vi "Main.vi"(11 "Module Admin":refnum<class "Delacor_lib_QMH_Module Admin.lvclass">) -> ()   [LabVIEW 2020, in "Config.lvlib"]
doc: "This template is based off of the Queued Message Handler design pattern and the Queued Message Handler project template that ships with LabVIEW.\n\nThe main difference is that the queue is private to this module and communication between modules is performed via Broadcast and Request events.\n\nRequest events are wrapped in public API methods and are handled in the Event Handling Loop (EHL) of this VI. Any module can register for Broadcast events sent by this module. The EHL generates messages based on user interface actions.\n\nThe Message Handling Loop (MHL) processes messages generated by the EHL, or by other messages. The messages are string values, so new messages can be added easily to the Message Cases case structure in the MHL. Each message cluster can also provide an optional value for Message Data, which is a variant that can be converted to whatever message-specific data is required.\n_____\nBased on Delacor QMH Project Template 5.0.0.82."
uses:
  Config.lvlib
  <vilib>/Delacor/Delacor QMH/Libraries/Module Admin_class/Delacor_lib_QMH_Module Admin.lvclass
  Module Data--cluster.ctl
  Stop Argument--cluster.ctl
  <vilib>/Delacor/Delacor QMH/Libraries/Message Queue_class/Delacor_lib_QMH_Message Queue.lvclass/Delacor_lib_QMH_Message Queue.ctl
  <vilib>/Delacor/Delacor QMH/Libraries/Module Admin_class/Delacor_lib_QMH_Module Admin.lvclass/Delacor_lib_QMH_Module Admin.ctl
  <vilib>/Utility/sysdir.llb/System Directory Type.ctl
  <vilib>/Delacor/Delacor QMH/Libraries/Message Queue_class/Delacor_lib_QMH_Enqueue Message (Single).vi
  <vilib>/Delacor/Delacor QMH/Libraries/Module Admin_class/Delacor_lib_QMH_Get External Launch.vi
  <vilib>/Utility/error.llb/Error Cluster From Error Code.vi
  <vilib>/ErrorRing/Error Ring.xnode
  <vilib>/Delacor/Delacor QMH/Libraries/Message Queue_class/Delacor_lib_QMH_Message Queue.lvclass
  Monedas/Monedas.lvlib
  Productos/Productos.lvlib
panel:
  in  "Productos":T1(array[cluster])
  in  "Monedas":cluster{"Valor":dbl, "Visible":bool}[](array[cluster])
  out "error out":errorcluster
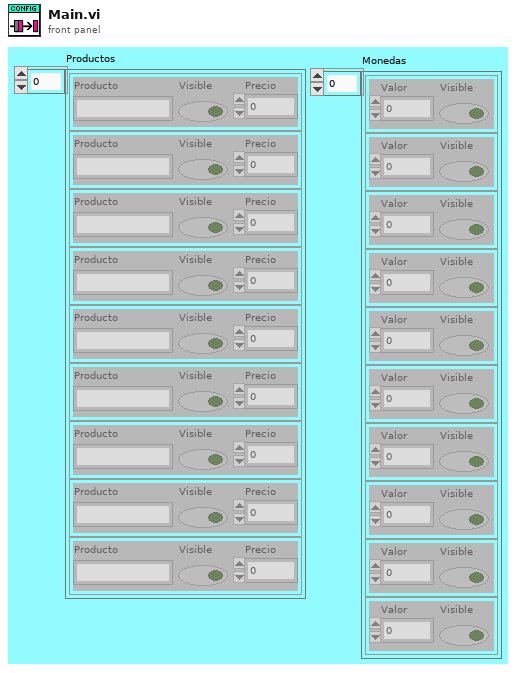
[diagram p1: front panel]
types:
  T1 = cluster{"Producto":string, "Visible":bool, "Precio":dbl}[]
  T2 = typedef "Config.lvlib/Request Events--cluster.ctl" = cluster{"Stop Module":refnum<user-event>, "Show Panel":refnum<user-event>, "Hide Panel":refnum<user-event>, "Get Module Execution Status":refnum<user-event>, "Show Diagram":refnum<user-event>}
  T3 = typedef "Config.lvlib/Module Data--cluster.ctl" = cluster{"Status":string}
  T4 = enum32{"invalid lock state", "Not Locked", "Locked (No Password)", "Password-protected"}
  T5 = typedef "Config.lvlib/Stop Argument--cluster.ctl" = cluster{"Origin":string, "Exit via Stop Module Req?":bool, "Wait for Module to stop?":bool}
  T6 = enum32{"Invalid", "Standard", "Closed", "Hidden", "Minimized", "Maximized"}
  T7 = enum16{"open", "replace", "create", "open or create", "replace or create", "replace or create with confirmation"}
  T8 = cluster{"Producto":string, "Boolean":bool, "Precio":dbl}[]
  T9 = typedef "System Directory Type.ctl" = i32
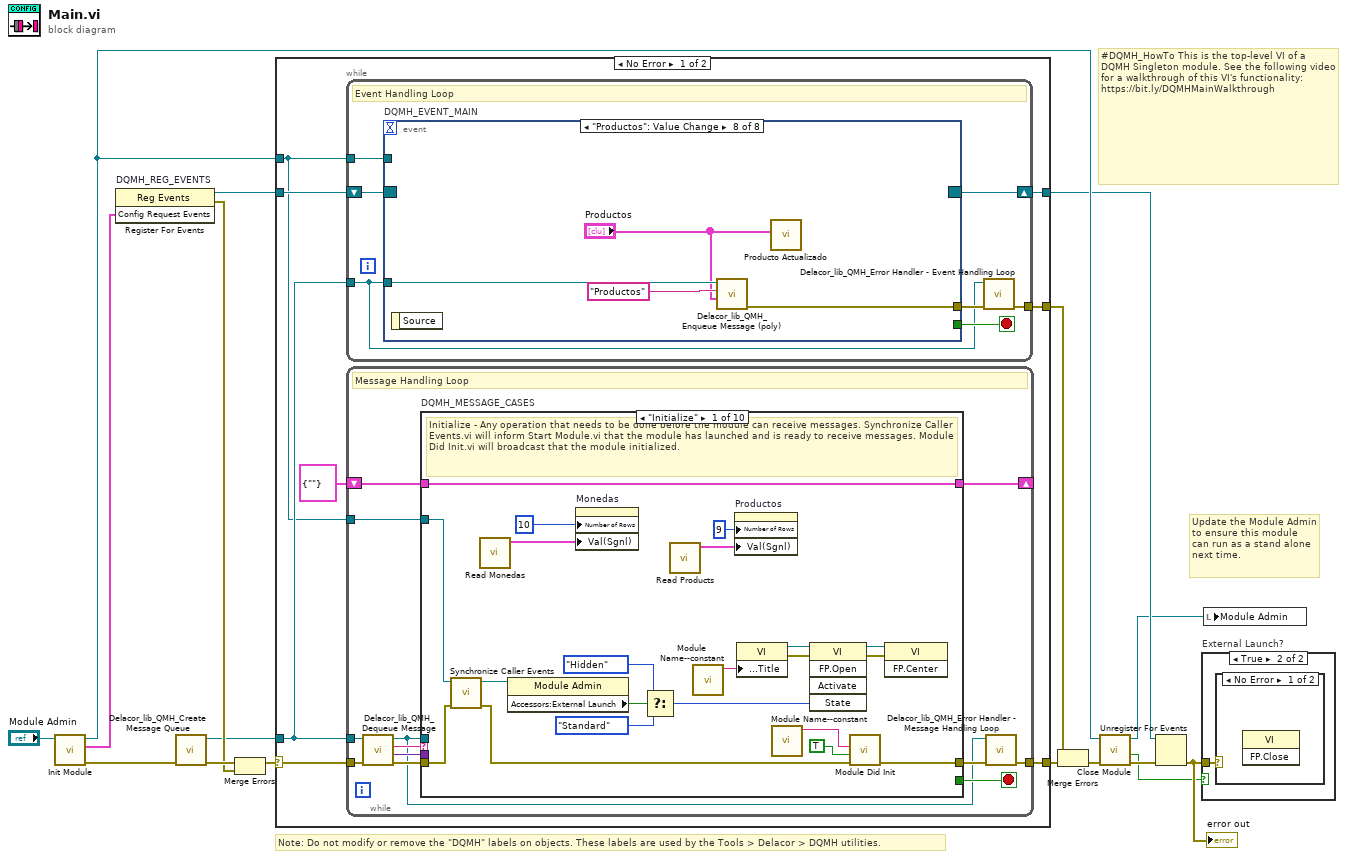
[diagram p0: block diagram]
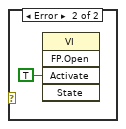
[diagram p3: hidden frame]
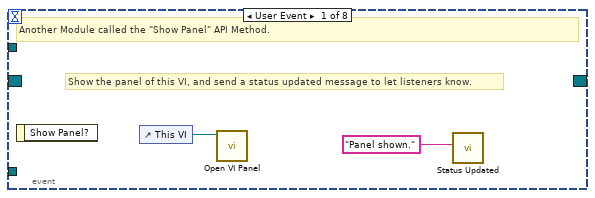
[diagram p4: hidden frame]
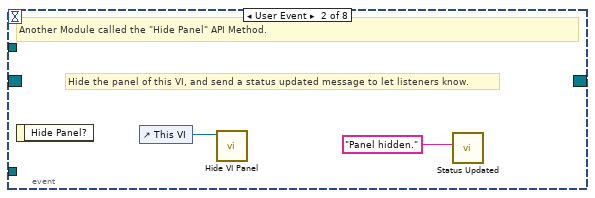
[diagram p5: hidden frame]
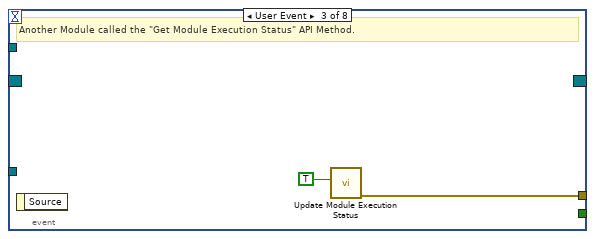
[diagram p6: hidden frame]
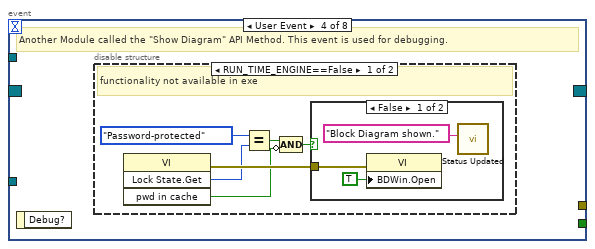
[diagram p7: hidden frame]
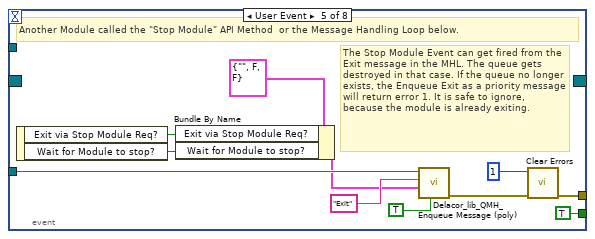
[diagram p10: hidden frame]
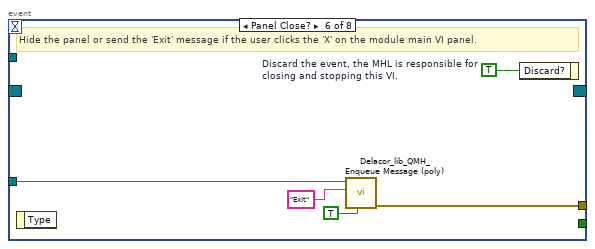
[diagram p11: hidden frame]
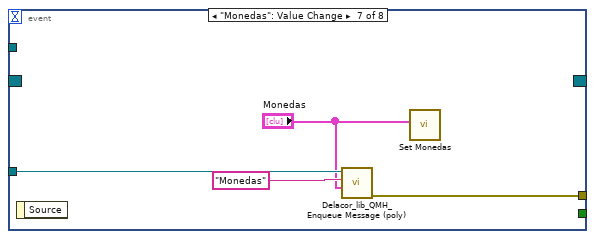
[diagram p12: hidden frame]
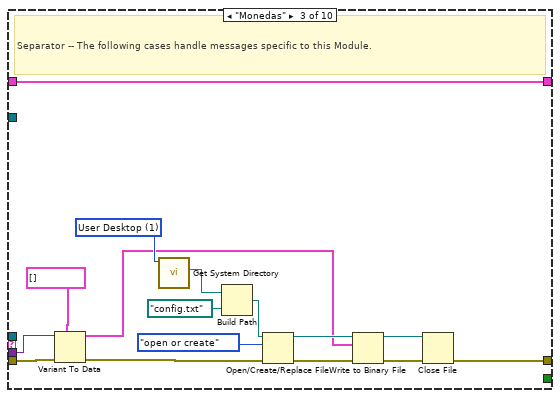
[diagram p14: hidden frame]
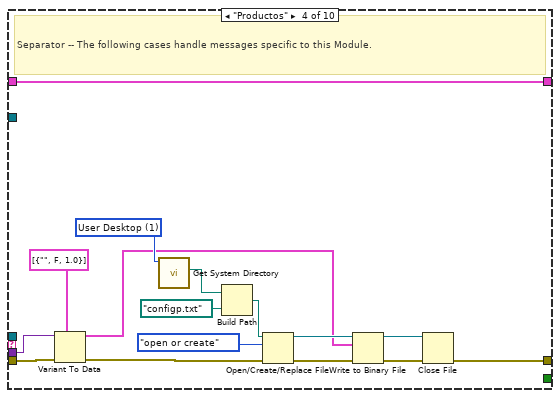
[diagram p15: hidden frame]
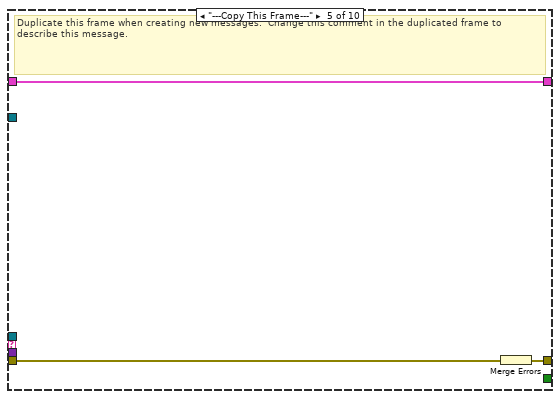
[diagram p16: hidden frame]
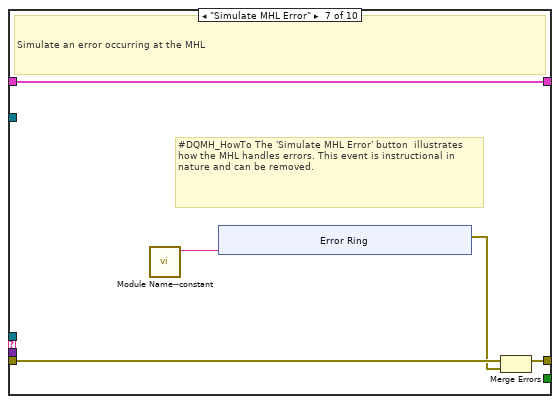
[diagram p18: hidden frame]
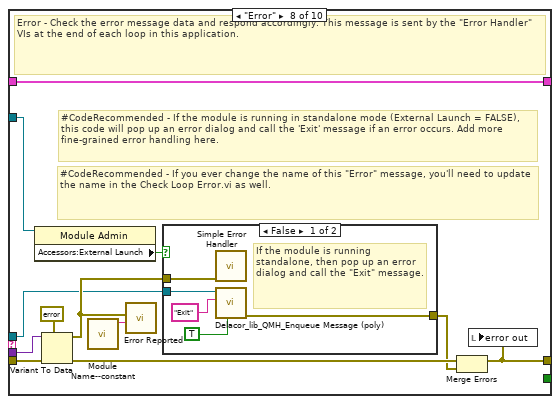
[diagram p19: hidden frame]
diagram:
  # "#DQMH_HowTo This is the top-level VI of a DQMH Singleton module. See the following video for a walkthrough of this VI's functionality: https://bit.ly/DQMHMainWalkthrough"
  # "Note: Do not modify or remove the \"DQMH\" labels on objects. These labels are used by the Tools > Delacor > DQMH utilities."
  # "Update the Module Admin to ensure this module can run as a stand alone next time."
  n1 = call "Init Module.vi"("Singleton Module Admin in"="Module Admin") -> ("error out"=w16:errorcluster, "Config Request Events"=w5:T2, "Singleton Module Admin out"=w8:refnum<class "Delacor_lib_QMH_Module Admin.lvclass">)  [unwired: 8 in]
  n2 = register-events "DQMH_REG_EVENTS"(w5) -> (reference out=w6:refnum<event-registration>, error out=w9:errorcluster)  [unwired: 2 in]
  n3 = call <vilib>:"Delacor_lib_QMH_Create Message Queue.vi"("error in (no error)"=w16) -> ("error out"=w11:errorcluster, "Message Queue"=w4:refnum<class "Delacor_lib_QMH_Message Queue.lvclass">)  [unwired: 9 in]
  n4 = Merge Errors(w11, w9) -> (w10:errorcluster)
  n5 = case shown="No Error" w10 {
    selector: w10 -> [w23 w204]
    tunnel: [w25 w203] -> w17
    tunnel: [w22 w209] -> w7
    tunnel: w6 -> [w20 w209]
    tunnel: w4 -> [w19 w202]
    tunnel: [w24 _] -> w14
    tunnel: w8 -> [w18 w205]
    frame No Error {
      n6 = while {
        tunnel: w19 -> [w26]
        shift-right: [w29] -> w22
        shift-left: w20 -> [w30]
        tunnel: [w31] -> w24
        tunnel: w18 -> [w27]
        stop <- w28 stop-if-true
        # "Event Handling Loop"
        n7 = event "DQMH_EVENT_MAIN" shown="[7] \"Productos\": Value Change" {
          selector: w30 -> [_ _ _ _ _ _ _ _]
          dyn-events: [_ _ _ _ _ _ _ _] -> w29
          timeout: _ -> [_ _ _ _ _ _ _ _]
          tunnel: [_ _ _ _ TRUE ("Discard?") _ _ _] -> w28
          tunnel: w26 -> [_ _ _ _ w54 w61 w66 w70]
          tunnel: [_ _ w38 _ w57 w63 w65 w69] -> w32
          tunnel: w27 -> [_ _ _ _ _ _ _ _]
          event User Event {
            # "Show the panel of this VI, and send a status updated message to let listeners know."
            # "Another Module called the \"Show Panel\" API Method."
            n8 = event-data() -> ()  [unwired: 1 in, 1 out]
            n9 = control-ref of="This VI"() -> (w34:refnum<vi>)
            n10 = call "Open VI Panel.vi"("VI"=w34) -> ()  [unwired: 10 in, 1 out]
            n11 = call "Status Updated.vi"("Status"="Panel shown." ("format string")) -> ()  [unwired: 10 in, 1 out]
          }
          event User Event {
            # "Hide the panel of this VI, and send a status updated message to let listeners know."
            # "Another Module called the \"Hide Panel\" API Method."
            n12 = event-data() -> ()  [unwired: 1 in, 1 out]
            n13 = control-ref of="This VI"() -> (w36:refnum<vi>)
            n14 = call "Hide VI Panel.vi"("VI"=w36) -> ()  [unwired: 10 in, 1 out]
            n15 = call "Status Updated.vi"("Status"="Panel hidden." ("format string")) -> ()  [unwired: 10 in, 1 out]
          }
          event User Event {
            # "Another Module called the \"Get Module Execution Status\" API Method."
            n16 = event-data() -> ()  [unwired: 1 in, 1 out]
            n17 = call "Update Module Execution Status.vi"("Running?"=TRUE) -> ("error out"=w38:errorcluster)  [unwired: 10 in]
          }
          event User Event {
            # "Another Module called the \"Show Diagram\" API Method. This event is used for debugging."
            n18 = event-data() -> ()  [unwired: 1 in, 1 out]
            n19 = disable-structure shown="RUN_TIME_ENGINE==False" {
              frame condition #0 (active) {
                # "functionality not available in exe"
                n20 = invoke class="VI" method="Lock State.Get"() -> (error out=w44:errorcluster, "Get Lock State"=w43:T4, "pwd in cache"=w40:bool)  [unwired: 4 in, 1 out]
                n21 = Equal?(x=T4."Password-protected", y=w43) -> (x = y?=w41:bool)
                n22 = Compound Arithmetic op=AND(w41, invert w40) -> (w39:bool)
                n23 = case shown="False" w39 {
                  tunnel: w44 -> [w47 _]
                  frame False {
                    n24 = property class="VI"(error in=w47, "BDWin.Open"=TRUE ("Block Diagram Window:Open")) -> ()  [unwired: 1 in, 2 out]
                    n25 = call "Status Updated.vi"("Status"="Block Diagram shown." ("format string")) -> ()  [unwired: 10 in, 1 out]
                  }
                  frame True {
                    # "Password-protected VI, and the password is not in the cache. Do not show the diagram."
                  }
                }
              }
              frame condition #1 {
              }
            }
          }
          event User Event {
            # "The Stop Module Event can get fired from the Exit message in the MHL. The queue gets destroyed in that case. If the queue no longer exists, the Enqueue Exit as a priority message will return error 1. It is safe to ignore, because the module is already exiting."
            # "Another Module called the \"Stop Module\" API Method  or the Message Handling Loop below."
            n26 = event-data() -> ("Exit via Stop Module Req?"=w50:bool, "Wait for Module to stop?"=w49:bool)  [unwired: 1 in]
            n27 = Bundle By Name(cluster=T5 {"Origin"="", "Exit via Stop Module Req?"=FALSE, "Wait for Module to stop?"=FALSE} ("Stop Argument"), "Exit via Stop Module Req?"=w50, "Wait for Module to stop?"=w49) -> (w48:T5)
            n28 = call-poly <vilib>:"Delacor_lib_QMH_Enqueue Message (poly).vi"("Priority Message? (F)"=TRUE, "Message Data"=w48, "Message"="Exit", "Message Queue in"=w54) -> ("error out"=w58:errorcluster)  [unwired: 6 in, 1 out]
            n29 = call <vilib>:"Clear Errors.vi"("error in (no error)"=w58, "specific error code to clear (0: all)"=1) -> ("error out"=w57:errorcluster)  [unwired: 4 in, 1 out]
          }
          event Panel Close? {
            w62 = TRUE  # Discard the event, the MHL is responsible for closing and stopping this VI.
            # "Hide the panel or send the 'Exit' message if the user clicks the 'X' on the module main VI panel."
            n30 = event-data() -> ()  [unwired: 1 in, 1 out]
            n31 = call-poly <vilib>:"Delacor_lib_QMH_Enqueue Message (poly).vi"("Priority Message? (F)"=TRUE, "Message"="Exit", "Message Queue in"=w61) -> ("error out"=w63:errorcluster)  [unwired: 7 in, 1 out]
            n32 = event-data("Discard?"=w62) -> ()  [unwired: 1 in, 1 out]
          }
          event "Monedas": Value Change {
            n33 = event-data() -> ()  [unwired: 1 in, 1 out]
            n34 = call-poly <vilib>:"Delacor_lib_QMH_Enqueue Message (poly).vi"("Message Data"="Monedas", "Message"="Monedas", "Message Queue in"=w66) -> ("error out"=w65:errorcluster)  [unwired: 7 in, 1 out]
            n35 = call "Set Monedas.vi"("Monedas"="Monedas") -> ()  [unwired: 10 in, 1 out]
          }
          event "Productos": Value Change {
            n36 = event-data() -> ()  [unwired: 1 in, 1 out]
            n37 = call-poly <vilib>:"Delacor_lib_QMH_Enqueue Message (poly).vi"("Message Data"="Productos", "Message"="Productos", "Message Queue in"=w70) -> ("error out"=w69:errorcluster)  [unwired: 7 in, 1 out]
            n38 = call "Producto Actualizado.vi"("Array"="Productos") -> ()  [unwired: 10 in, 1 out]
          }
        }
        n39 = call-dynamic "Delacor_lib_QMH_Error Handler - Event Handling Loop.vi"("error in (no error)"=w32, "Message Queue in"=w26) -> ("dup error in"=w31:errorcluster)  [unwired: 8 in, 1 out]
      }
      n40 = while {
        tunnel: w19 -> [w74]
        shift-right: [w78] -> _
        shift-left: T3 {"Status"=""} ("Data Cluster") -> [w79]
        tunnel: w23 -> [w82]
        tunnel: [w80] -> w25
        tunnel: w18 -> [w72]
        stop <- w77 stop-if-true
        # "Message Handling Loop"
        n41 = call-dynamic "Delacor_lib_QMH_Dequeue Message.vi"("error in (no error)"=w82, "Message Queue in"=w74) -> ("error out"=w81:errorcluster, "Message Data"=w75:variant, "Message"=w76:string, "Message Queue out"=w73:refnum<class "Delacor_lib_QMH_Message Queue.lvclass">)  [unwired: 6 in]
        n42 = case "DQMH_MESSAGE_CASES" shown="\"Initialize\"" w76 {
          selector: w76 -> [_ _ _ _ _ _ _ _ _ w189]
          tunnel: w73 -> [_ _ _ _ _ _ _ w159 w181 _]
          tunnel: w81 -> [w102 w106 w113 w129 w141 w143 w148 w166 w187 w191]
          tunnel: [w100 w106 w112 w128 w140 w143 w147 w162 w184 w192] -> w83
          tunnel: w79 -> [w91 w105 w122 w138 w139 w142 w145 w161 w180 w190]
          tunnel: [w91 w105 w122 w138 w139 w142 w145 w161 w180 w190] -> w78
          tunnel: [_ _ _ _ _ _ _ _ w179 _] -> w77
          tunnel: w75 -> [_ _ w109 w125 _ _ _ w160 w178 _]
          tunnel: w72 -> [w92 _ _ _ _ _ _ w158 w173 _]
          frame "Initialize" {
            # "Initialize - Any operation that needs to be done before the module can receive messages. Synchronize Caller Events.vi will inform Start Module.vi that the module has launched and is ready to receive messages. Module Did Init.vi will broadcast that the module initialized."
            n43 = call "Synchronize Caller Events.vi"("error in (no error)"=w102, "Singleton Module Admin in"=w92) -> ("error out"=w101:errorcluster, "Singleton Module Admin out"=w88:refnum<class "Delacor_lib_QMH_Module Admin.lvclass">)  [unwired: 8 in]
            n44 = call "Read Monedas.vi"() -> ("Array"=w86:cluster{"Numeric":dbl, "Boolean":bool}[])  [unwired: 10 in, 1 out]
            n45 = property class="Module Admin"(reference=w88) -> ("Accessors:External Launch"=w96:bool)  [unwired: 1 in, 2 out]
            n46 = property on="Monedas" class="Arr (strict)"("Number of Rows"=u32 10 ("Number of Columns"), "Val(Sgnl)"=w86) -> ()  [unwired: 2 in, 2 out]
            n47 = Select(t=T6."Hidden" ("State"), s=w96, f=T6."Standard" ("State")) -> (s? t:f=w93:T6)
            n48 = call "Read Products.vi"() -> ("Array"=w84:T8)  [unwired: 10 in, 1 out]
            n49 = call "Module Name--constant.vi"() -> ("Module Name"=w99:string)  [unwired: 11 in]
            n50 = property on="Productos" class="Arr (strict)"("Number of Rows"=u32 9, "Val(Sgnl)"=w84) -> ()  [unwired: 2 in, 2 out]
            n51 = property class="VI"("Front Panel.Title"=w99) -> (reference out=w98:refnum<vi>, error out=w104:errorcluster)  [unwired: 2 in]
            n52 = call "Module Name--constant.vi"() -> ("Module Name"=w89:string)  [unwired: 11 in]
            n53 = invoke class="VI" method="FP.Open"(reference=w98, error in=w104, "State"=w93) -> (reference out=w97:refnum<vi>, error out=w103:errorcluster)  [unwired: 2 in, 3 out]
            n54 = call "Module Did Init.vi"("error in (no error)"=w101, "Initialized?"=TRUE, "Origin"=w89) -> ("error out"=w100:errorcluster)  [unwired: 8 in]
            n55 = invoke class="VI" method="FP.Center"(reference=w97, error in=w103) -> ()  [unwired: 1 in, 3 out]
          }
          frame "--- Module Specific ---" {
            # "Separator -- The following cases handle messages specific to this Module."
          }
          frame "Monedas" {
            w111 = T9 1 items=["User Home"=0, "User Desktop"=1, "User Documents"=2, "User Application Data"=3, "User Preferences"=4, "User Temporary"=5, "Public Documents"=6, "Public Application Data"=7, "Public Preferences"=8, "Public Cache"=13, "System Core Libraries"=9, "System Installed Libraries"=10, "Application Files"=11, "Boot Volume Root"=12] ("system directory type")
            # "Separator -- The following cases handle messages specific to this Module."
            n56 = Variant To Data(error in=w113, type=cluster{"Numeric":dbl, "Boolean":bool}[] [] ("Monedas"), Variant=w109) -> (data=w107:cluster{"Numeric":dbl, "Boolean":bool}[], error out=w110:errorcluster)
            n57 = call <vilib>:"Get System Directory.vi"("system directory type"=w111) -> ("system directory"=w119:path)  [unwired: 10 in]
            n58 = Build Path(base path=w119, name or relative path=path "config.txt") -> (appended path=w117:path)
            n59 = Open/Create/Replace File(file path (use dialog)=w117, error in=w110, operation (0:open)=T7."open or create") -> (refnum out=w121:refnum<file>, error out=w116:errorcluster)  [unwired: 3 in, 1 out]
            n60 = Write to Binary File(file (use dialog)=w121, data=w107, error in=w116) -> (refnum out=w114:refnum<file>, error out=w115:errorcluster)  [unwired: 3 in, 1 out]
            n61 = Close File(refnum=w114, error in=w115) -> (error out=w112:errorcluster)  [unwired: 1 out]
          }
          frame "Productos" {
            w127 = T9 1 items=["User Home"=0, "User Desktop"=1, "User Documents"=2, "User Application Data"=3, "User Preferences"=4, "User Temporary"=5, "Public Documents"=6, "Public Application Data"=7, "Public Preferences"=8, "Public Cache"=13, "System Core Libraries"=9, "System Installed Libraries"=10, "Application Files"=11, "Boot Volume Root"=12] ("system directory type")
            # "Separator -- The following cases handle messages specific to this Module."
            n62 = Variant To Data(error in=w129, type=T1 [{"Producto"="", "Visible"=FALSE, "Precio"=1.0}] ("Productos"), Variant=w125) -> (data=w124:T1, error out=w126:errorcluster)
            n63 = call <vilib>:"Get System Directory.vi"("system directory type"=w127) -> ("system directory"=w135:path)  [unwired: 10 in]
            n64 = Build Path(base path=w135, name or relative path=path "configp.txt") -> (appended path=w133:path)
            n65 = Open/Create/Replace File(file path (use dialog)=w133, error in=w126, operation (0:open)=T7."open or create") -> (refnum out=w137:refnum<file>, error out=w132:errorcluster)  [unwired: 3 in, 1 out]
            n66 = Write to Binary File(file (use dialog)=w137, data=w124, error in=w132) -> (refnum out=w130:refnum<file>, error out=w131:errorcluster)  [unwired: 3 in, 1 out]
            n67 = Close File(refnum=w130, error in=w131) -> (error out=w128:errorcluster)  [unwired: 1 out]
          }
          frame "---Copy This Frame---" {
            # "Duplicate this frame when creating new messages.  Change this comment in the duplicated frame to describe this message."
            n68 = Merge Errors(w141) -> (w140:errorcluster)
          }
          frame "--- Exit and Error Handling---" {
            # "Separator - The following cases handle errors and exit messages."
          }
          frame "Simulate MHL Error" {
            # "#DQMH_HowTo The 'Simulate MHL Error' button  illustrates how the MHL handles errors. This event is instructional in nature and can be removed."
            # "Simulate an error occurring at the MHL"
            n69 = call "Module Name--constant.vi"() -> ("Module Name"=w144:string)  [unwired: 11 in]
            n70 = xnode "Error Ring"("parameter 0"=w144) -> ("error out"=w146:errorcluster)
            n71 = Merge Errors(w148, w146) -> (w147:errorcluster)
          }
          frame "Error" {
            # "#CodeRecommended - If you ever change the name of this \"Error\" message, you'll need to update the name in the Check Loop Error.vi as well."
            # "#CodeRecommended - If the module is running in standalone mode (External Launch = FALSE), this code will pop up an error dialog and call the 'Exit' message if an error occurs. Add more fine-grained error handling here."
            # "Error - Check the error message data and respond accordingly. This message is sent by the \"Error Handler\" VIs at the end of each loop in this application."
            n72 = property class="Module Admin"(reference=w158) -> ("Accessors:External Launch"=w157:bool)  [unwired: 1 in, 2 out]
            n73 = Variant To Data(error in=w166, type=errorcluster {"status"=FALSE, "code"=0, "source"=""} ("error constant"), Variant=w160) -> (data=w167:errorcluster, error out=w164:errorcluster)
            n74 = call "Module Name--constant.vi"() -> ("Module Name"=w156:string)  [unwired: 11 in]
            n75 = call "Error Reported.vi"("Additional Information"=w156, "Error"=w167) -> ()  [unwired: 9 in, 1 out]
            n76 = case shown="False" w157 {
              tunnel: [w172 _] -> w163
              tunnel: w159 -> [w170 _]
              tunnel: w167 -> [w171 _]
              frame False {
                # "If the module is running standalone, then pop up an error dialog and call the \"Exit\" message."
                n77 = call <vilib>:"Simple Error Handler.vi"("error in (no error)"=w171) -> ()  [unwired: 4 in, 5 out]
                n78 = call-poly <vilib>:"Delacor_lib_QMH_Enqueue Message (poly).vi"("Priority Message? (F)"=TRUE, "Message"="Exit", "Message Queue in"=w170) -> ("error out"=w172:errorcluster)  [unwired: 7 in, 1 out]
              }
              frame True {
                # "If the module was launched externally, calling the Error Reported broadcast VI is the only action performed by the \"Error\" message. The module's caller can then process the error appropriately."
              }
            }
            n79 = Merge Errors(w164, w163) -> (w162:errorcluster)
            n80 = local write "error out"(w162) -> ()
          }
          frame "Exit" {
            w177 = 91  # 91: not all Exit messages will have an argument
            w179 = TRUE  # Stop the VI
            # "Release the message queue reference"
            # "#CodeNeeded - Add any required cleanup code here"
            # "Exit - Exit the application."
            n81 = Variant To Data(error in=w187, type=T5 {"Origin"="", "Exit via Stop Module Req?"=FALSE, "Wait for Module to stop?"=FALSE} ("Stop Argument"), Variant=w178) -> (data=w175:T5, error out=w183:errorcluster)
            n82 = call <vilib>:"Clear Errors.vi"("error in (no error)"=w183, "specific error code to clear (0: all)"=w177) -> ("error out"=w186:errorcluster)  [unwired: 4 in, 1 out]
            n83 = control-ref of="This VI"() -> (w174:refnum<vi>)
            n84 = call-dynamic "Delacor_lib_QMH_Release Message Queue.vi"("error in (no error)"=w186, "Message Queue"=w181) -> ("error out"=w185:errorcluster)  [unwired: 9 in]
            n85 = call "Handle Exit.vi"("Stop Argument"=w175, "Admin in"=w173, "VI reference"=w174) -> ("error out"=w182:errorcluster)  [unwired: 7 in, 1 out]
            n86 = Merge Errors(w185, w182) -> (w184:errorcluster)
          }
          frame Default {
            # "'Default' case only runs if there is a message that isn't defined in any of the other cases.  Output a programming error."
            n87 = call "Module Name--constant.vi"() -> ("Module Name"=w188:string)  [unwired: 11 in]
            n88 = xnode "Error Ring"("parameter 0"=w189, "parameter 1"=w188) -> ("error out"=w193:errorcluster)
            n89 = Merge Errors(w191, w193) -> (w192:errorcluster)
          }
        }
        n90 = call-dynamic "Delacor_lib_QMH_Error Handler - Message Handling Loop.vi"("error in (no error)"=w83, "Message Queue in"=w73) -> ("dup error in"=w80:errorcluster)  [unwired: 8 in, 1 out]
      }
    }
    frame Error {
      # "Synchronize Caller Events.vi will inform Start Module.vi that the module has launched and will let the code calling Start Module.vi register for broadcasts and would permit the caller receive the broadcast that an error occurred at launch time."
      n91 = call-dynamic "Delacor_lib_QMH_Release Message Queue.vi"("error in (no error)"=w204, "Message Queue"=w202) -> ("error out"=w203:errorcluster)  [unwired: 9 in]
      n92 = call "Synchronize Caller Events.vi"("Singleton Module Admin in"=w205) -> ("error out"=w210:errorcluster)  [unwired: 9 in, 1 out]
      n93 = call "Module Name--constant.vi"() -> ("Module Name"=w208:string)  [unwired: 11 in]
      n94 = Format Into String(format string="An error occurred during initialization. %s is no longer running.", w208) -> (resulting string=w206:string)  [unwired: 2 in, 1 out]
      n95 = Merge Errors(w203, w210) -> (w211:errorcluster)
      n96 = call "Error Reported.vi"("Additional Information"=w206, "Error"=w211) -> ()  [unwired: 9 in, 1 out]
    }
  }
  n97 = Merge Errors(w14, w17) -> (w13:errorcluster)
  n98 = call "Close Module.vi"("error in (no error)"=w13, "Module Admin in"=w8) -> ("error out"=w15:errorcluster, "External Launch"=w1:bool, "Module Admin out"=w2:refnum<class "Delacor_lib_QMH_Module Admin.lvclass">)  [unwired: 7 in]
  n99 = Unregister For Events(event registration refnum=w7, error in=w15) -> (error out=w12:errorcluster)
  "error out" <- w12
  n100 = case "External Launch?" shown="True" w1 {
    tunnel: w12 -> [_ w212]
    frame False {
    }
    frame True {
      n101 = case shown="No Error" w212 {
        frame No Error {
          n102 = invoke class="VI" method="FP.Close"() -> ()  [unwired: 3 in, 3 out]
        }
        frame Error {
          n103 = invoke class="VI" method="FP.Open"("Activate"=TRUE ("Activate?")) -> ()  [unwired: 4 in, 5 out]
        }
      }
    }
  }
  n104 = local write "Module Admin"(w2) -> ()
